vi "Wirst Set Position.vi"(7 "Description":string, 8 "Command Info In":T1, 11 "Setpoint (Degrees)":dbl) -> (0 "Command Info Out":T1)   [LabVIEW 2018]
doc: "This template is useful for immediate subsystem actions that do not need deadband filtering\n\nBe sure to right-click and select New from Template and save with a new command name."
uses:
  <vilib>/Rock Robotics/WPI/Framework/Command Status Info.ctl
  <vilib>/Rock Robotics/WPI/Framework/Completion Status.ctl
  <vilib>/Rock Robotics/WPI/Framework/Completion Notifier.ctl
  Implementation/Wrist Setpoints.ctl
  Implementation/Wrist Operations.ctl
  Beak/Implementation/Beak Published Globals.vi
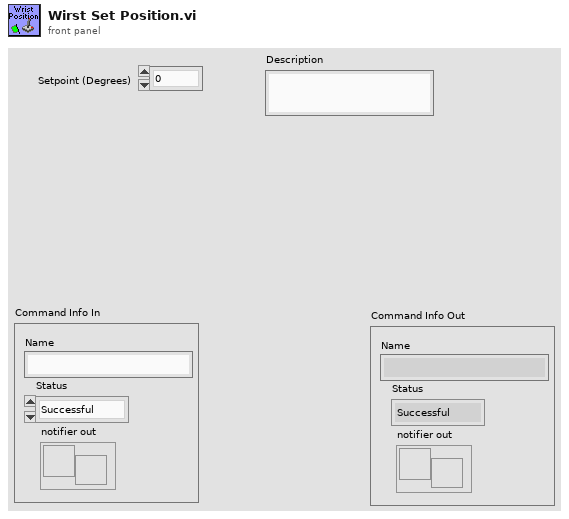
[diagram p1: front panel]
types:
  T1 = typedef "Command Status Info.ctl" = cluster{"Name":string, "Status":T2, "notifier out":T3}
  T2 = typedef "Completion Status.ctl" = enum16{"Successful", "Aborted", "Incomplete"}
  T3 = typedef "Completion Notifier.ctl" = refnum<notifier>
  T4 = typedef "Wrist Setpoints.ctl" = cluster{"Operation":T5, "Setpoint":dbl, "Duration":dbl}
  T5 = typedef "Wrist Operations.ctl" = enum16{"Reserve", "Read Current", "Immediate", "Set Position"}
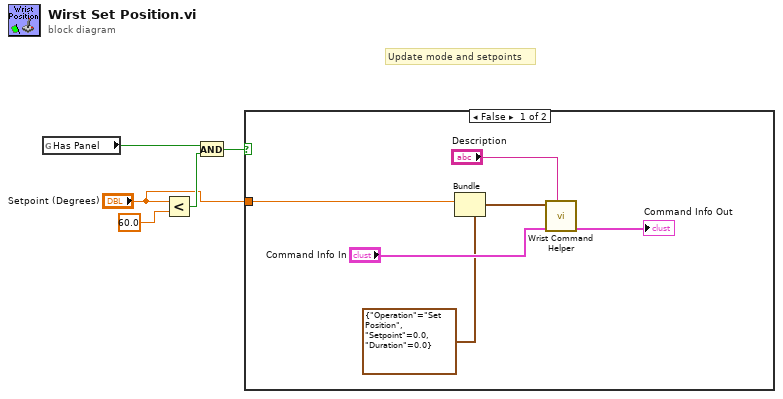
[diagram p0: block diagram]
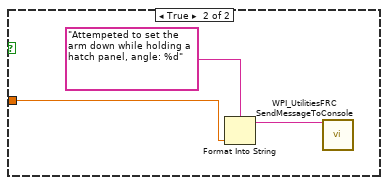
[diagram p2: hidden frame]
diagram:
  # "Update mode and setpoints"
  n1 = global read "Beak Published Globals.vi" "Has Panel"() -> (w3:bool)
  n2 = Less?(x="Setpoint (Degrees)", y=60.0) -> (x < y?=w4:bool)
  n3 = And(x=w3, y=w4) -> (x .and. y?=w2:bool)
  n4 = case shown="False" w2 {
    tunnel: "Setpoint (Degrees)" -> [w6 w13]
    frame False {
      n5 = Bundle(cluster=T4 {"Operation"=enum."Set Position", "Setpoint"=0.0, "Duration"=0.0} ("SubSystem Data"), "Setpoint"=w6) -> (w7:T4)  [unwired: 2 in]
      n6 = call "Wrist Command Helper.vi"("Description"="Description", "Command Info In"="Command Info In", "SubSystem Data"=w7) -> ("Command Info Out"=→"Command Info Out":T1)  [unwired: 6 in, 2 out]
    }
    frame True {
      n7 = Format Into String(format string="Attempeted to set the arm down while holding a hatch panel, angle: %d" ("Message"), w13) -> (resulting string=w12:string)  [unwired: 2 in, 1 out]
      n8 = call <vilib>:"WPI_UtilitiesFRC SendMessageToConsole.vi"("Message"=w12) -> ()  [unwired: 14 in, 1 out]
    }
  }
